vi "Load CSV.vi"() -> (10 "Header":string[](array[string]), 11 "error out":errorcluster, 12 "CSV Array":string[][](array[string]), 13 "indices":T1, 14 "Fuel":string[](array[string]), 15 "Oxidizer":string[](array[string]), 16 "Initial Pressure":string[](array[string]), 17 "Equivalence Ratio":string[](array[string]), 18 "Diluent":string[](array[string]), 19 "Diluent Mole Fraction":string[](array[string]))   [LabVIEW 2018]
uses:
  <vilib>/Utility/file.llb/Read Delimited Spreadsheet (string).vi
  Sort 1D Array sub vis/Sort 1D String.vi
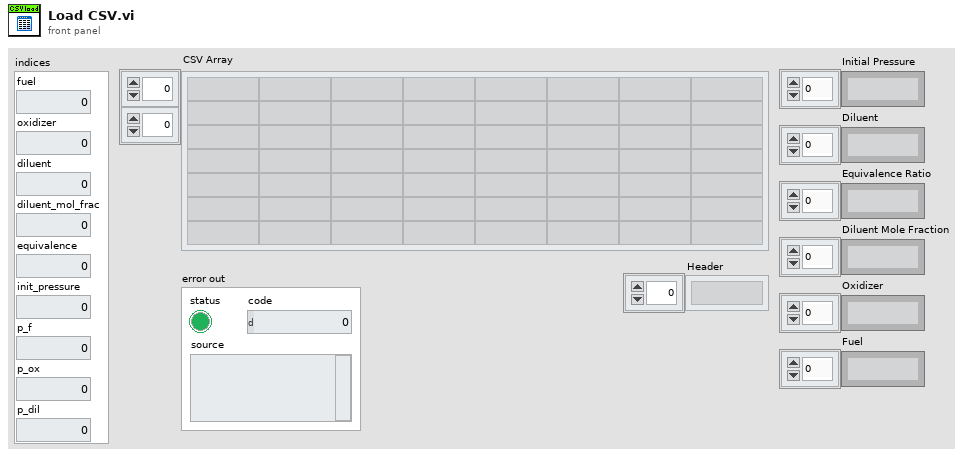
[diagram p1: front panel]
types:
  T1 = cluster{"fuel":i32, "oxidizer":i32, "diluent":i32, "diluent_mol_frac":i32, "equivalence":i32, "init_pressure":i32, "p_f":i32, "p_ox":i32, "p_dil":i32}
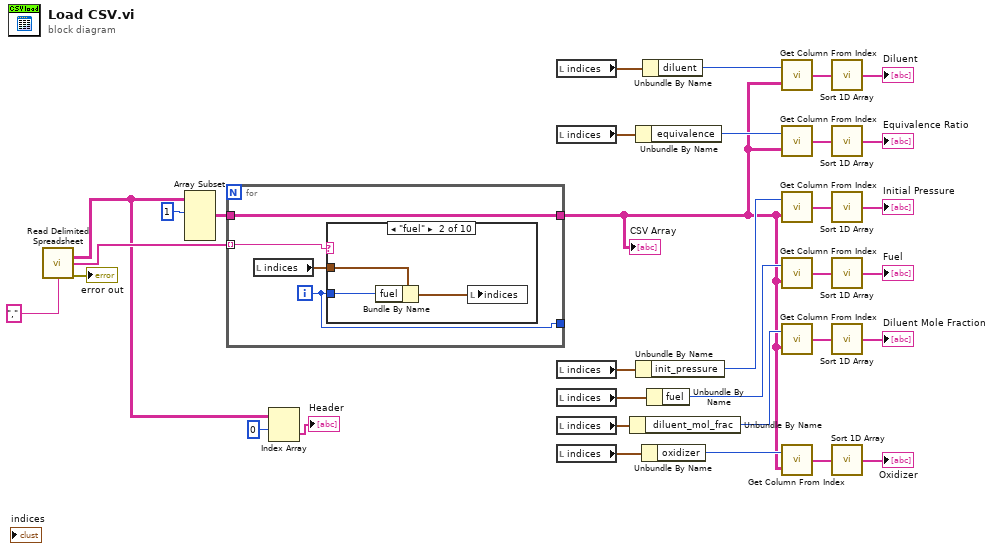
[diagram p0: block diagram]
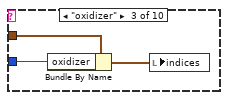
[diagram p3: hidden frame]
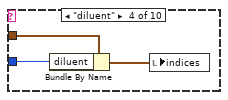
[diagram p4: hidden frame]
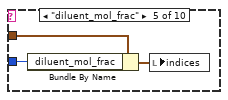
[diagram p5: hidden frame]
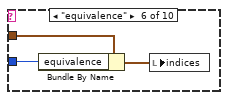
[diagram p6: hidden frame]
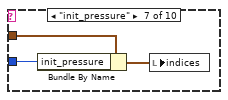
[diagram p7: hidden frame]
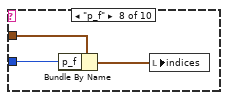
[diagram p8: hidden frame]
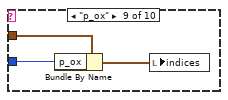
[diagram p9: hidden frame]
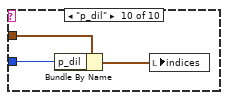
[diagram p10: hidden frame]
diagram:
  n1 = call-poly <vilib>:"Read Delimited Spreadsheet.vi"("delimiter (\\t)"="," ("delimiter (\\t)")) -> ("all rows"=w3:string[][], "first row"=w31:string[], "error out"=→"error out":errorcluster)  [unwired: 9 in, 3 out]
  n2 = Array Subset(array=w3, index (row)=1 ("index")) -> (w27:string[][])  [unwired: 3 in]
  n3 = for {
    tunnel: w31 -> [w37] mode=indexing
    tunnel: [w36] -> _
    tunnel: w27 -> [w34]
    tunnel: [w34] -> w11
    i -> [w36]
    n4 = local read "indices"() -> (w35:T1)
    n5 = case shown="\"fuel\"" w37 {
      tunnel: w35 -> [_ w40 w41 w44 w48 w51 w53 w57 w59 w62]
      tunnel: w36 -> [_ w39 w43 w45 w47 w50 w54 w56 w60 w63]
      frame Default {
      }
      frame "fuel" {
        n6 = Bundle By Name(cluster=w40, "fuel"=w39) -> (w38:T1)
        n7 = local write "indices"(w38) -> ()
      }
      frame "oxidizer" {
        n8 = Bundle By Name(cluster=w41, "oxidizer"=w43) -> (w42:T1)
        n9 = local write "indices"(w42) -> ()
      }
      frame "diluent" {
        n10 = Bundle By Name(cluster=w44, "diluent"=w45) -> (w46:T1)
        n11 = local write "indices"(w46) -> ()
      }
      frame "diluent_mol_frac" {
        n12 = Bundle By Name(cluster=w48, "diluent_mol_frac"=w47) -> (w49:T1)
        n13 = local write "indices"(w49) -> ()
      }
      frame "equivalence" {
        n14 = Bundle By Name(cluster=w51, "equivalence"=w50) -> (w52:T1)
        n15 = local write "indices"(w52) -> ()
      }
      frame "init_pressure" {
        n16 = Bundle By Name(cluster=w53, "init_pressure"=w54) -> (w55:T1)
        n17 = local write "indices"(w55) -> ()
      }
      frame "p_f" {
        n18 = Bundle By Name(cluster=w57, "p_f"=w56) -> (w58:T1)
        n19 = local write "indices"(w58) -> ()
      }
      frame "p_ox" {
        n20 = Bundle By Name(cluster=w59, "p_ox"=w60) -> (w61:T1)
        n21 = local write "indices"(w61) -> ()
      }
      frame "p_dil" {
        n22 = Bundle By Name(cluster=w62, "p_dil"=w63) -> (w64:T1)
        n23 = local write "indices"(w64) -> ()
      }
    }
  }
  "CSV Array" <- w11
  n24 = Index Array(array=w3, index (row)=0) -> (element=→"Header":string[])  [unwired: 1 in]
  n25 = local read "indices"() -> (w22:T1)
  n26 = local read "indices"() -> (w19:T1)
  n27 = local read "indices"() -> (w25:T1)
  n28 = local read "indices"() -> (w29:T1)
  n29 = local read "indices"() -> (w16:T1)
  n30 = local read "indices"() -> (w13:T1)
  n31 = Unbundle By Name(w16) -> ("diluent_mol_frac"=w15:i32)
  n32 = Unbundle By Name(w19) -> ("equivalence"=w20:i32)
  n33 = Unbundle By Name(w25) -> ("init_pressure"=w26:i32)
  n34 = Unbundle By Name(w13) -> ("oxidizer"=w14:i32)
  n35 = Unbundle By Name(w22) -> ("diluent"=w21:i32)
  n36 = Unbundle By Name(w29) -> ("fuel"=w28:i32)
  n37 = call "Get Column From Index.vi"("array"=w11, "index"=w21) -> ("subarray"=w23:string[])
  n38 = call "Get Column From Index.vi"("array"=w11, "index"=w20) -> ("subarray"=w18:string[])
  n39 = call "Get Column From Index.vi"("array"=w11, "index"=w26) -> ("subarray"=w24:string[])
  n40 = call "Get Column From Index.vi"("array"=w11, "index"=w28) -> ("subarray"=w30:string[])
  n41 = call "Get Column From Index.vi"("array"=w11, "index"=w15) -> ("subarray"=w17:string[])
  n42 = call "Get Column From Index.vi"("array"=w11, "index"=w14) -> ("subarray"=w12:string[])
  n43 = call-poly "Sort 1D Array.vi"("1D input array"=w23) -> ("output array"=→"Diluent":string[])
  n44 = call-poly "Sort 1D Array.vi"("1D input array"=w18) -> ("output array"=→"Equivalence Ratio":string[])
  n45 = call-poly "Sort 1D Array.vi"("1D input array"=w24) -> ("output array"=→"Initial Pressure":string[])
  n46 = call-poly "Sort 1D Array.vi"("1D input array"=w30) -> ("output array"=→"Fuel":string[])
  n47 = call-poly "Sort 1D Array.vi"("1D input array"=w17) -> ("output array"=→"Diluent Mole Fraction":string[])
  n48 = call-poly "Sort 1D Array.vi"("1D input array"=w12) -> ("output array"=→"Oxidizer":string[])
